vi "Generate Event.vi"(10 "PS4 Controller in":T2 {"R2" scale=-32768.0..32767.0; "L2" scale=-32768.0..32767.0}, 11 "Event Ref":T1) -> ()   [LabVIEW 2021]
uses:
  <vilib>/MakerHub/PS4-Controller/Private/Type Defs/Indicators/Controller.ctl
  <vilib>/MakerHub/PS4-Controller/Private/Type Defs/Indicators/Square.ctl
  <vilib>/MakerHub/PS4-Controller/Private/Type Defs/Indicators/X.ctl
  <vilib>/MakerHub/PS4-Controller/Private/Type Defs/Indicators/Circle.ctl
  <vilib>/MakerHub/PS4-Controller/Private/Type Defs/Indicators/Triangle.ctl
  <vilib>/MakerHub/PS4-Controller/Private/Type Defs/Indicators/L1.ctl
  <vilib>/MakerHub/PS4-Controller/Private/Type Defs/Indicators/R1.ctl
  <vilib>/MakerHub/PS4-Controller/Private/Type Defs/Indicators/Share.ctl
  <vilib>/MakerHub/PS4-Controller/Private/Type Defs/Indicators/Options.ctl
  <vilib>/MakerHub/PS4-Controller/Private/Type Defs/Indicators/PS.ctl
  <vilib>/MakerHub/PS4-Controller/Private/Type Defs/Indicators/Pad_Button.ctl
  <vilib>/MakerHub/PS4-Controller/Private/Type Defs/Indicators/Dpad.ctl
  <vilib>/MakerHub/PS4-Controller/Private/Type Defs/Indicators/Slider.ctl
  event cluster.ctl
  <vilib>/MakerHub/PS4-Controller/LMH-PS4.lvlib
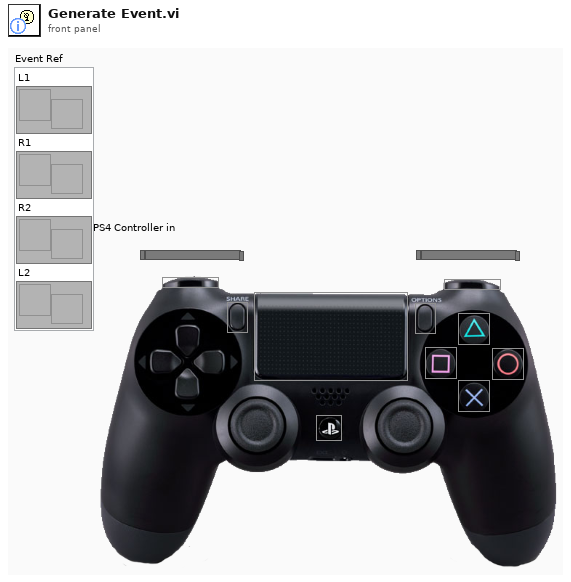
[diagram p1: front panel]
types:
  T1 = typedef "event cluster.ctl" = cluster{"L1":refnum<user-event>, "R1":refnum<user-event>, "R2":refnum<user-event>, "L2":refnum<user-event>}
  T2 = typedef "LMH-PS4.lvlib/Controller.ctl" = cluster{"Square Button":T3, "X Button":T4, "Circle Button":T5, "Triangle Button":T6, "L1":T7, "R1":T8, "Share Button":T9, "Options Button":T10, "PS Button":T11, "Pad Button":T12, "D-Pad":T13, "L2":T14, "R2":T14, "Thumbstick_Left":cluster{i32[], i32[]}, "Thumbstick_Right":cluster{i32[], i32[]}}
  T3 = typedef "LMH-PS4.lvlib/Square.ctl" = bool
  T4 = typedef "LMH-PS4.lvlib/X.ctl" = bool
  T5 = typedef "LMH-PS4.lvlib/Circle.ctl" = bool
  T6 = typedef "LMH-PS4.lvlib/Triangle.ctl" = bool
  T7 = typedef "LMH-PS4.lvlib/L1.ctl" = bool
  T8 = typedef "LMH-PS4.lvlib/R1.ctl" = bool
  T9 = typedef "LMH-PS4.lvlib/Share.ctl" = bool
  T10 = typedef "LMH-PS4.lvlib/Options.ctl" = bool
  T11 = typedef "LMH-PS4.lvlib/PS.ctl" = bool
  T12 = typedef "LMH-PS4.lvlib/Pad_Button.ctl" = bool
  T13 = typedef "LMH-PS4.lvlib/Dpad.ctl" = u16
  T14 = typedef "LMH-PS4.lvlib/Slider.ctl" = i32
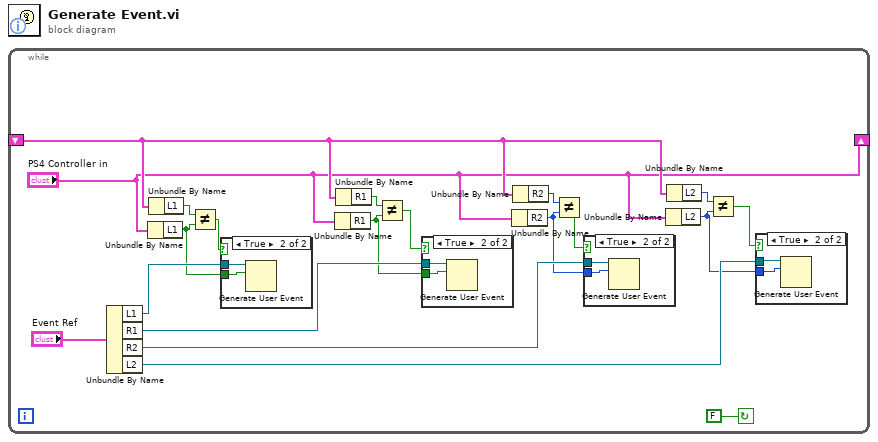
[diagram p0: block diagram]
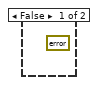
[diagram p2: hidden frame]
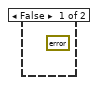
[diagram p3: hidden frame]
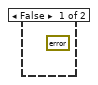
[diagram p4: hidden frame]
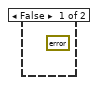
[diagram p5: hidden frame]
diagram:
  n1 = while {
    shift-right: ["PS4 Controller in"] -> _
    shift-left: _ -> [w3]
    stop <- FALSE continue-if-true
    n2 = Unbundle By Name("Event Ref") -> ("L1"=w18:refnum<user-event>, "R1"=w14:refnum<user-event>, "R2"=w7:refnum<user-event>, "L2"=w5:refnum<user-event>)
    n3 = Unbundle By Name("PS4 Controller in") -> ("L1"=w15:T7)
    n4 = Unbundle By Name(w3) -> ("L1"=w17:T7)
    n5 = Not Equal?(x=w17, y=w15) -> (x != y?=w16:T7)
    n6 = case shown="True" w16 {
      tunnel: w18 -> [_ w28]
      tunnel: w15 -> [_ w27]
      frame False {
        (unwired) errorcluster {"status"=FALSE, "code"=0, "source"=""} ("error out")
      }
      frame True {
        n7 = Generate User Event(user event=w28, event data cluster=w27) -> ()  [unwired: 2 in, 2 out]
      }
    }
    n8 = Unbundle By Name("PS4 Controller in") -> ("R1"=w11:T8)
    n9 = Unbundle By Name(w3) -> ("R1"=w13:T8)
    n10 = Not Equal?(x=w13, y=w11) -> (x != y?=w12:T8)
    n11 = case shown="True" w12 {
      tunnel: w14 -> [_ w26]
      tunnel: w11 -> [_ w25]
      frame False {
        (unwired) errorcluster {"status"=FALSE, "code"=0, "source"=""} ("error out")
      }
      frame True {
        n12 = Generate User Event(user event=w26, event data cluster=w25) -> ()  [unwired: 2 in, 2 out]
      }
    }
    n13 = Unbundle By Name("PS4 Controller in") -> ("R2"=w6:T14)
    n14 = Unbundle By Name(w3) -> ("R2"=w9:T14)
    n15 = Not Equal?(x=w9, y=w6) -> (x != y?=w8:bool)
    n16 = case shown="True" w8 {
      tunnel: w7 -> [_ w24]
      tunnel: w6 -> [_ w23]
      frame False {
        (unwired) errorcluster {"status"=FALSE, "code"=0, "source"=""} ("error out")
      }
      frame True {
        n17 = Generate User Event(user event=w24, event data cluster=w23) -> ()  [unwired: 2 in, 2 out]
      }
    }
    n18 = Unbundle By Name("PS4 Controller in") -> ("L2"=w1:T14)
    n19 = Unbundle By Name(w3) -> ("L2"=w10:T14)
    n20 = Not Equal?(x=w10, y=w1) -> (x != y?=w4:bool)
    n21 = case shown="True" w4 {
      tunnel: w5 -> [_ w22]
      tunnel: w1 -> [_ w21]
      frame False {
        (unwired) errorcluster {"status"=FALSE, "code"=0, "source"=""} ("error out")
      }
      frame True {
        n22 = Generate User Event(user event=w22, event data cluster=w21) -> ()  [unwired: 2 in, 2 out]
      }
    }
  }
